vi "Extract Unlabeled Data.vi"() -> ()   [LabVIEW 2013]
uses:
  <vilib>/Utility/file.llb/Write To Spreadsheet File (DBL).vi
panel:
  out "Currently Processing:":string
  out "Progress":u8(slide) scale=0.0..100.0
  out "error out":errorcluster
  in  "error in (no error)":errorcluster
  in  "Sample File":path
  in  "AVI Directory":path
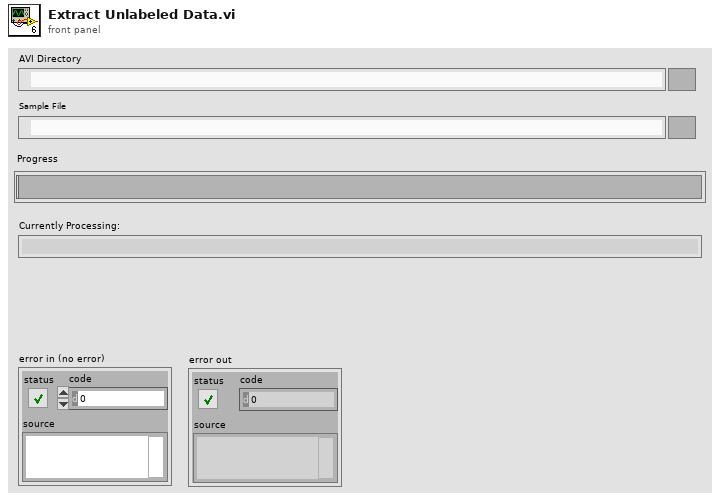
[diagram p1: front panel]
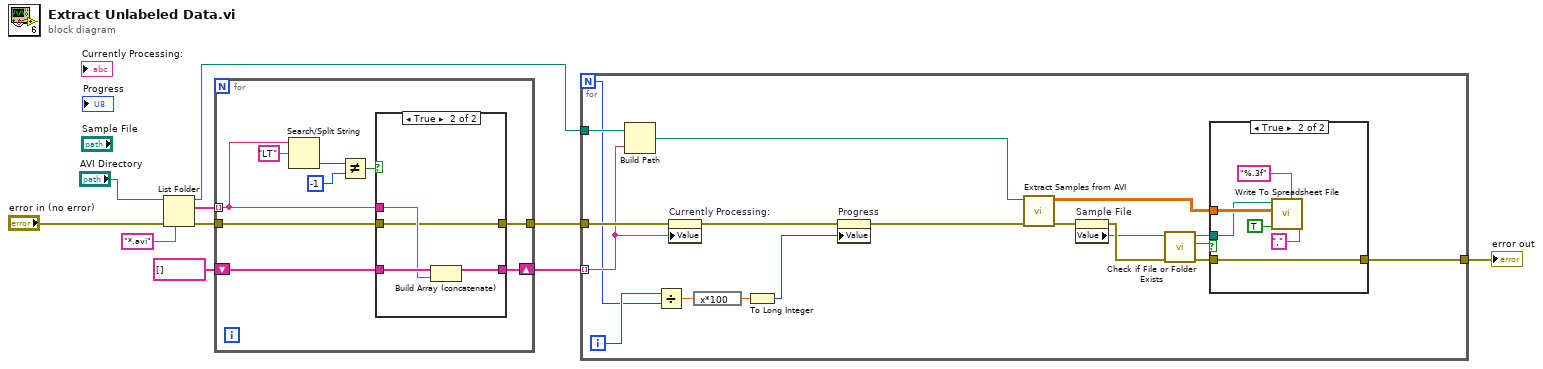
[diagram p0: block diagram]
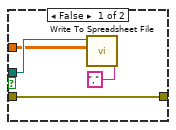
[diagram p2: hidden frame]
diagram:
  n1 = List Folder(path="AVI Directory", pattern="*.avi", error in="error in (no error)") -> (path out=w3:path, filenames=w8:string[], error out=w7:errorcluster)  [unwired: 1 in, 1 out]
  n2 = for {
    tunnel: w8 -> [w13] mode=indexing
    tunnel: w7 -> [w12]
    shift-right: [w14] -> w4
    shift-left: string[] [] -> [w15]
    tunnel: [w11] -> w2
    n3 = Search/Split String(string=w13, search string/char (-)="LT") -> (offset of match=w19:i32)  [unwired: 1 in, 2 out]
    n4 = Not Equal?(x=w19, y=-1) -> (x != y?=w16:bool)
    n5 = case shown="True" w16 {
      tunnel: w15 -> [w20 w25]
      tunnel: [w20 w24] -> w14
      tunnel: w13 -> [_ w23]
      tunnel: w12 -> [w21 w22]
      tunnel: [w21 w22] -> w11
      frame False {
      }
      frame True {
        n6 = Build Array (concatenate)(w25, w23) -> (w24:string[])
      }
    }
  }
  n7 = for {
    N -> [w30]
    tunnel: w4 -> [w33] mode=indexing
    tunnel: w3 -> [w44]
    tunnel: w2 -> [w34]
    tunnel: [w35] -> w1
    i -> [w31]
    n8 = Build Path(base path=w44, name or relative path=w33) -> (appended path=w43:path)
    n9 = Divide(x=w31, y=w30) -> (x/y=w29:dbl)
    n10 = property on="Currently Processing:" class="Str"(error in=w34, "Value"=w33) -> (error out=w32:errorcluster)  [unwired: 1 in, 1 out]
    n11 = expression code="x*100"(w29) -> (w28:dbl)
    n12 = To Long Integer(number=w28) -> (32bit integer=w27:i32)
    n13 = property on="Progress" class="Slide (strict)"(error in=w32, "Value"=w27) -> (error out=w26:errorcluster)  [unwired: 1 in, 1 out]
    n14 = call "Extract Samples from AVI.vi"("error in (no error)"=w26, "AVI Path"=w43) -> ("error out"=w42:errorcluster, "Samples"=w41:dbl[][])  [unwired: 8 in]
    n15 = property on="Sample File" class="Path"(error in=w42) -> (error out=w40:errorcluster, "Value"=w39:path)  [unwired: 1 in, 1 out]
    n16 = call <vilib>:"Check if File or Folder Exists.vi"("error in (no error)"=w40, "path"=w39) -> ("error out"=w37:errorcluster, "file or folder exists?"=w38:bool, "dup path"=w36:path)  [unwired: 7 in]
    n17 = case shown="True" w38 {
      tunnel: w41 -> [w46 w52]
      tunnel: w37 -> [w47 w50]
      tunnel: w36 -> [w48 w51]
      tunnel: [w47 w50] -> w35
      frame False {
        n18 = call-poly <vilib>:"Write To Spreadsheet File.vi"("delimiter (\\t)"="," ("delimiter (\\t)"), "2D data"=w46, "file path (dialog if empty)"=w48) -> ()  [unwired: 5 in, 1 out]
      }
      frame True {
        n19 = call-poly <vilib>:"Write To Spreadsheet File.vi"("delimiter (\\t)"="," ("delimiter (\\t)"), "format (%.3f)"="%.3f", "append to file? (new file:F)"=TRUE, "2D data"=w52, "file path (dialog if empty)"=w51) -> ()  [unwired: 3 in, 1 out]
      }
    }
  }
  "error out" <- w1
